vi "Listen_close.vi"(8 "error in (no error)":errorcluster, 11 "Socket.TCP in":refnum<class "Socket.TCP.lvclass">) -> (0 "error out":errorcluster, 3 "Socket.TCP out":refnum<class "Socket.TCP.lvclass">)   [LabVIEW 2014, in "Socket.lvlib" / "Socket.TCP.lvclass"]
doc: "Closes the listener. \n\nMust run after Listen_wait has attached or timed out and before running Listen again."
uses:
  Socket.TCP.lvclass
  Socket.TCP.lvclass/Socket.TCP.ctl
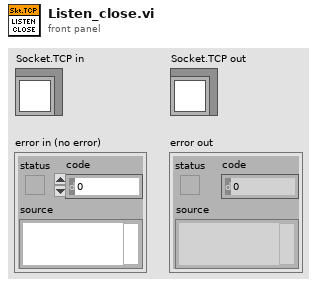
[diagram p1: front panel]
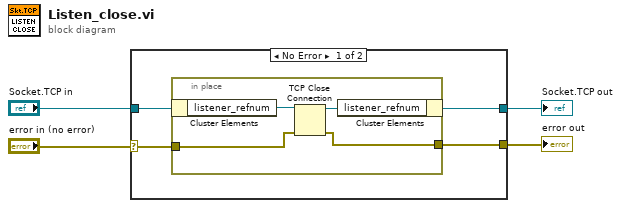
[diagram p0: block diagram]
diagram:
  n1 = case shown="No Error" "error in (no error)" {
    selector: "error in (no error)" -> [w7 w14]
    tunnel: [w6 w14] -> w3
    tunnel: [w5 w13] -> w1
    tunnel: "Socket.TCP in" -> [w8 w13]
    frame No Error {
      n2 = in-place {
        in-place-border: w7 -> [w10]
        in-place-border: [w9] -> w6
        n3 = in-place-cluster #1(w8) -> ("listener_refnum"=w12:refnum<k5>)
        n4 = TCP Close Connection(connection ID=w12, error in (no error)=w10) -> (connection ID out=w11:refnum<k5>, error out=w9:errorcluster)  [unwired: 1 in]
        n5 = in-place-cluster #1("listener_refnum"=w11) -> (w5:refnum<class "Socket.TCP.lvclass">)
      }
    }
    frame Error {
    }
  }
  "error out" <- w3
  "Socket.TCP out" <- w1
